vi "ShowMinMaxOn Graoh.vi"(5 "Log Mode?":bool, 7 "WaveformGraph in":refnum<vi>, 10 "Range (Vpp)":dbl, 11 "output waveform":cluster{"Start Time":dbl, dbl, ext[]}) -> (0 "max index Log":i32, 1 "Max Log":ext, 2 "Time (sec)":dbl, 3 "Max Abs":ext)   [LabVIEW 2020]
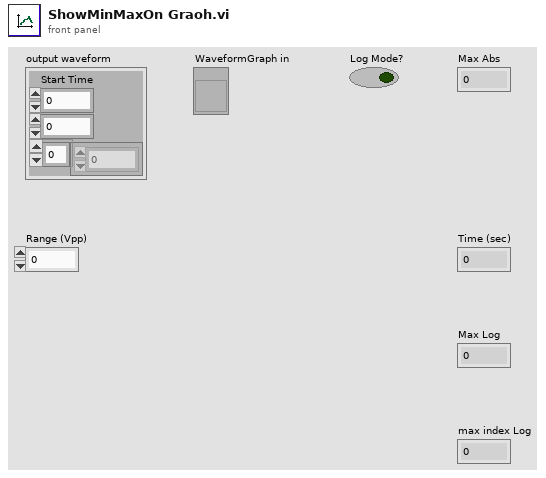
[diagram p1: front panel]
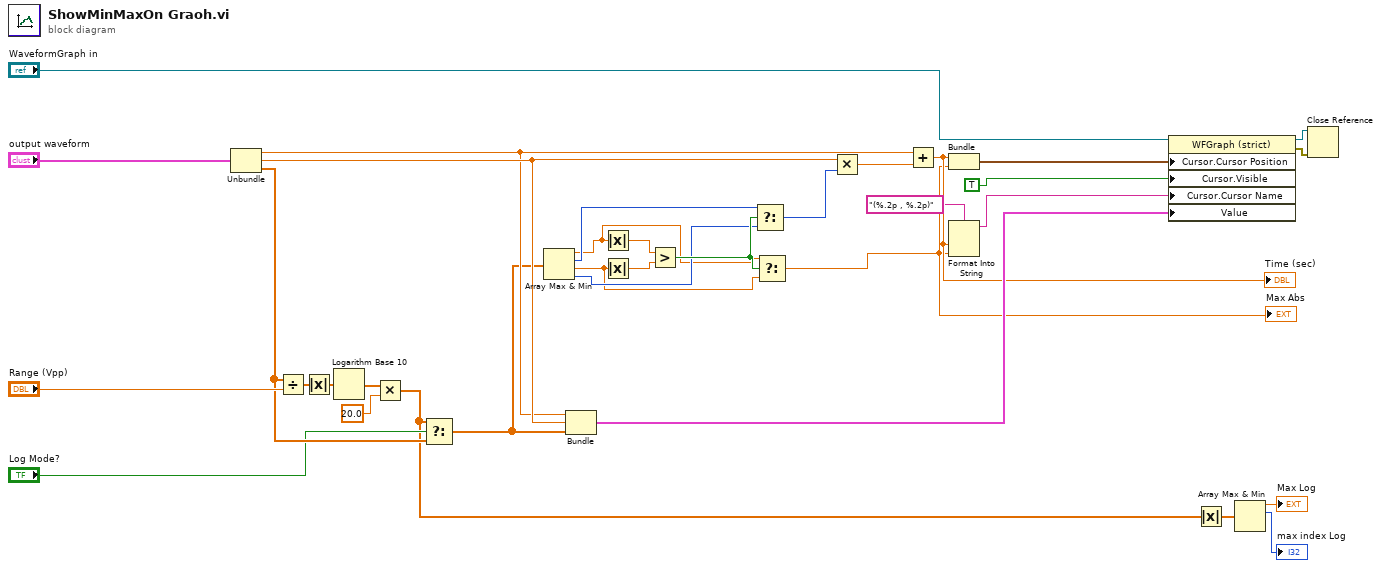
[diagram p0: block diagram]
diagram:
  n1 = Unbundle("output waveform") -> ("Start Time"=w31:dbl, w32:dbl, w30:ext[])
  n2 = Divide(x=w30, y="Range (Vpp)") -> (x/y=w27:ext[])
  n3 = Absolute Value(x=w27) -> (abs(x)=w26:ext[])
  n4 = Logarithm Base 10(1:w26) -> (0:w29:ext[])
  n5 = Multiply(x=w29, y=20.0 ("Sample Rate")) -> (x*y=w6:ext[])
  n6 = Select(t=w6, s="Log Mode?", f=w30) -> (s? t:f=w16:ext[])
  n7 = Array Max & Min(array=w16) -> (max value=w8:ext, max index (indices)=w10:i32, min value=w7:ext, min index (indices)=w9:i32)
  n8 = Bundle("Start Time"=w31, w32, w16) -> (w33:cluster{"Start Time":dbl, dbl, ext[]})  [unwired: 1 in]
  n9 = Absolute Value(x=w8) -> (abs(x)=w15:ext)
  n10 = Absolute Value(x=w7) -> (abs(x)=w14:ext)
  n11 = Greater?(x=w15, y=w14) -> (0:w11:bool)
  n12 = Select(t=w10, s=w11, f=w9) -> (s? t:f=w12:i32)
  n13 = Select(t=w8, s=w11, f=w7) -> (s? t:f=w13:ext)
  "Max Abs" <- w13
  n14 = Multiply(x=w32, y=w12) -> (x*y=w20:dbl)
  n15 = Add(x=w31, y=w20) -> (x+y=w22:dbl)
  "Time (sec)" <- w22
  n16 = Bundle(w22, w13) -> (w17:cluster{dbl, ext})  [unwired: 1 in]
  n17 = Format Into String(format string="(%.2p , %.2p)", w22, w13) -> (resulting string=w23:string)  [unwired: 2 in, 1 out]
  n18 = property on="Property Node" class="WFGraph (strict)"(reference="WaveformGraph in", "Cursor.Cursor Position"=w17, "Cursor.Visible"=TRUE, "Cursor.Cursor Name"=w23, "Value"=w33) -> (reference out=w2:refnum<vi>, error out=w1:errorcluster)  [unwired: 1 in]
  n19 = Absolute Value(x=w6) -> (abs(x)=w5:ext[])
  n20 = Array Max & Min(array=w5) -> (max value=→"Max Log":ext, max index (indices)=→"max index Log":i32)  [unwired: 2 out]
  n21 = Close Reference(reference=w2, error in (no error)=w1) -> ()  [unwired: 1 out]
